vi "A33ReadError.vi"() -> ()   [LabVIEW 2022 SP3]
panel:
  out "Response":string
  out "error out":errorcluster
  in  "VISA resource name":refnum<visa-resource-name>
  in  "error in (no error)":errorcluster
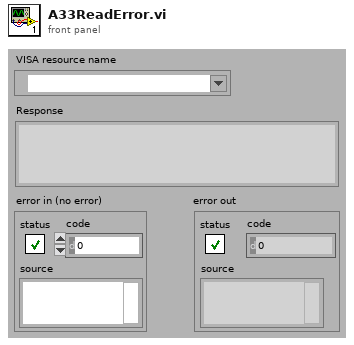
[diagram p1: front panel]
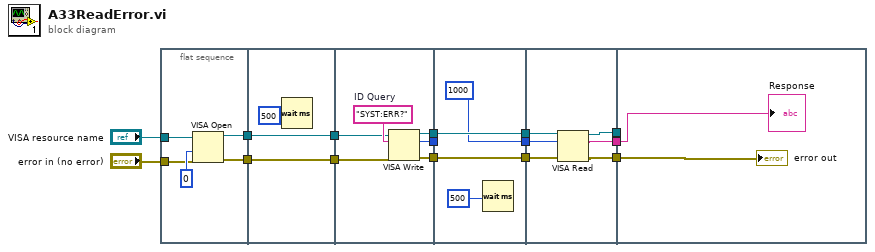
[diagram p0: block diagram]
diagram:
  n1 = flat-sequence {
    tunnel: [w18] -> w9
    tunnel: [w19] -> w8
    tunnel: "VISA resource name" -> [w17]
    tunnel: "error in (no error)" -> [w16]
    tunnel: [w23] -> w2
    tunnel: [w22] -> w1
    tunnel: w9 -> [w22]
    tunnel: w8 -> [w23]
    tunnel: [w29] -> w15
    tunnel: [w28] -> w14
    tunnel: [w24] -> w13
    tunnel: w2 -> [w26]
    tunnel: w1 -> [w25]
    tunnel: w15 -> [w33]
    tunnel: w14 -> [w32]
    tunnel: w13 -> [_]
    tunnel: [w33] -> w12
    tunnel: [w32] -> w11
    tunnel: [u32 1000] -> w10
    tunnel: w12 -> [w39]
    tunnel: w11 -> [w37]
    tunnel: w10 -> [w38]
    tunnel: [w36] -> w5
    tunnel: [w35] -> w4
    tunnel: [w34] -> w3
    tunnel: w5 -> [w40]
    tunnel: w4 -> [w41]
    tunnel: w3 -> [_]
    frame #0 {
      n2 = VISA Open(access mode=u32 0, error in (no error)=w16, VISA resource name=w17) -> (VISA resource name=w19:refnum<visa-resource-name>, error out=w18:errorcluster)  [unwired: 2 in]
    }
    frame #1 {
      n3 = Wait (ms)(milliseconds to wait=u32 500) -> ()  [unwired: 1 out]
    }
    frame #2 {
      w27 = "SYST:ERR?"  # ID Query
      n4 = VISA Write(VISA resource name=w26, write buffer=w27, error in (no error)=w25) -> (VISA resource name out=w29:refnum<visa-resource-name>, return count=w24:u32, error out=w28:errorcluster)
    }
    frame #3 {
      n5 = Wait (ms)(milliseconds to wait=u32 500) -> ()  [unwired: 1 out]
    }
    frame #4 {
      n6 = VISA Read(VISA resource name=w39, byte count=w38, error in (no error)=w37) -> (VISA resource name out=w34:refnum<visa-resource-name>, read buffer=w35:string, error out=w36:errorcluster)  [unwired: 1 out]
    }
    frame #5 {
      "error out" <- w40
      "Response" <- w41
    }
  }
